vi "shutter all shutters.vi"   [LabVIEW 2011]
doc: "This vi is intended to be a stand-alone executable, to be invoked by a logon script, tha tputs the lasers in a safe state before they are powered up."
uses:
  h-nu-ixon/Laser type.ctt
types:
  T1 = typedef "Laser type.ctt" = enum16{"Blue 488 nm", "Green 532 nm", "Orange 594 nm", "Red 633 nm", "IR 780"}
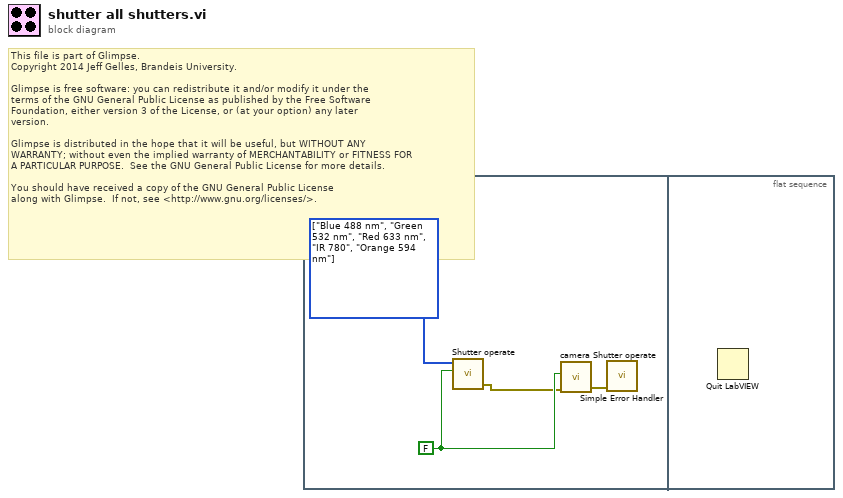
[diagram p0: block diagram]
diagram:
  # "This file is part of Glimpse. \nCopyright 2014 Jeff Gelles, Brandeis University.    \n\nGlimpse is free software: you can redistribute it and/or modify it under the \nterms of the GNU General Public License as published by the Free Software \nFoundation, either version 3 of the License, or (at your option) any later \nversion.\n\nGlimpse is distributed in the hope that it will be useful, but WITHOUT ANY \nWARRANTY; without even the implied warranty of MERCHANTABILITY or FITNESS FOR \nA PARTICULAR PURPOSE.  See the GNU General Public License for more details.\n\nYou should have received a copy of the GNU General Public License\nalong with Glimpse.  If not, see <http://www.gnu.org/licenses/>."
  n1 = flat-sequence {
    frame #0 {
      w4 = T1[] [enum."Blue 488 nm", enum."Green 532 nm", enum."Red 633 nm", enum."IR 780", enum."Orange 594 nm"] items=["Blue 488 nm", "Green 532 nm", "Orange 594 nm", "Red 633 nm", "IR 780"] ("Shutters")
      w3 = FALSE
      n2 = call "Shutter operate.vi"("Shutters"=w4, 2:w3) -> ("error out"=w2:errorcluster)  [unwired: 1 in, 5 out]
      n3 = call "camera Shutter operate.vi"("Open?"=w3, "error in"=w2) -> ("error out"=w1:errorcluster)  [unwired: 6 in]
      n4 = call <vilib>:"Simple Error Handler.vi"("error in (no error)"=w1) -> ()  [unwired: 4 in, 5 out]
    }
    frame #1 {
      n5 = Quit LabVIEW() -> ()  [unwired: 1 in]
    }
  }
